vi "SetScanParams.vi"(6 "ScanFunc":i32, 7 "DescKword":string, 8 "error in":errorcluster, 9 "Experiment.lvclass":refnum<class "Experiment.lvclass">, 10 "SinglePar":bool, 11 "Interface.lvclass":refnum<class "Interface.lvclass">) -> (0 "error out":errorcluster, 1 "Experiment.lvclass Out":refnum<class "Experiment.lvclass">, 2 "DataFileName":path, 3 "Interface.lvclass Out":refnum<class "Interface.lvclass">, 4 "Scan list":string[](array[string]), 5 "DataFileRef":refnum<file>)   [LabVIEW 2019, in "Interface.lvclass"]
doc: "Ce Vi prend les données d'acquisition et les formatte en tableau de \"string\" pour ensuite les sauvegarder sous le format .txt"
uses:
  Interface.lvclass
  Experiment Class/Experiment.lvclass
  Interface.lvclass/Interface.ctl
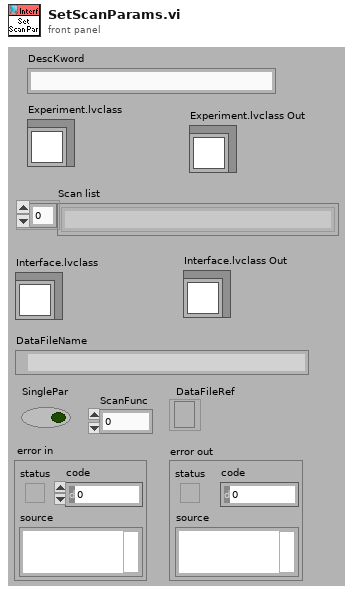
[diagram p1: front panel]
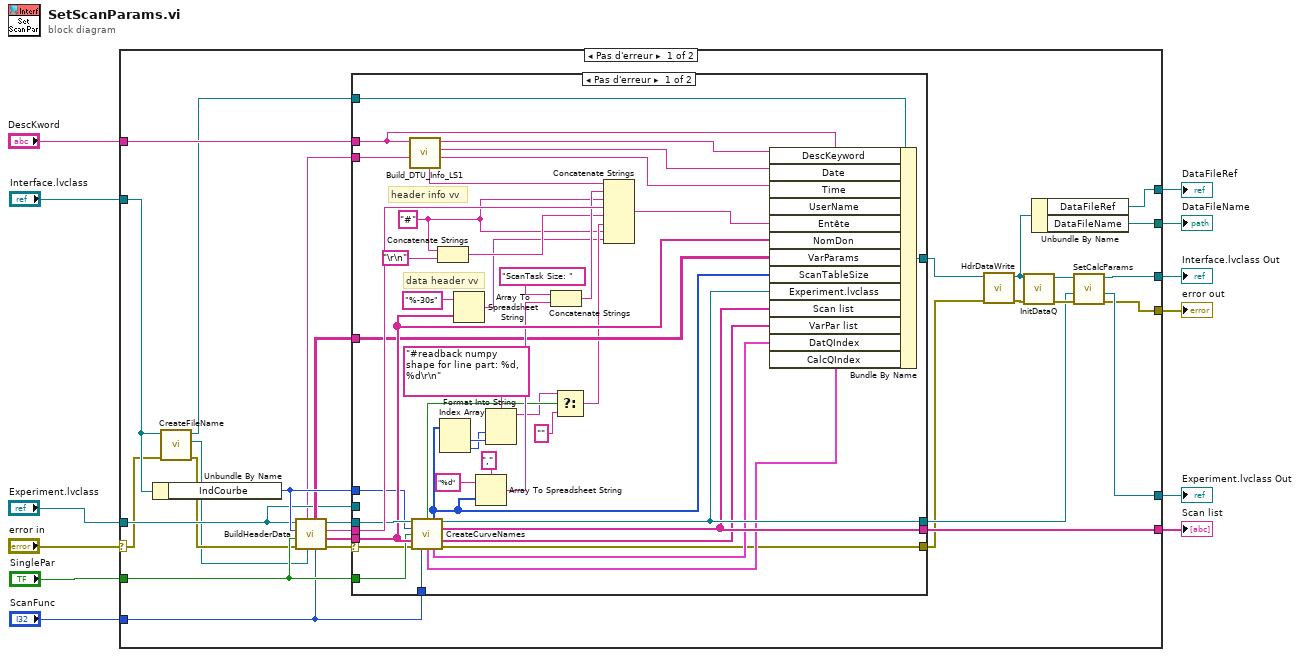
[diagram p0: block diagram]
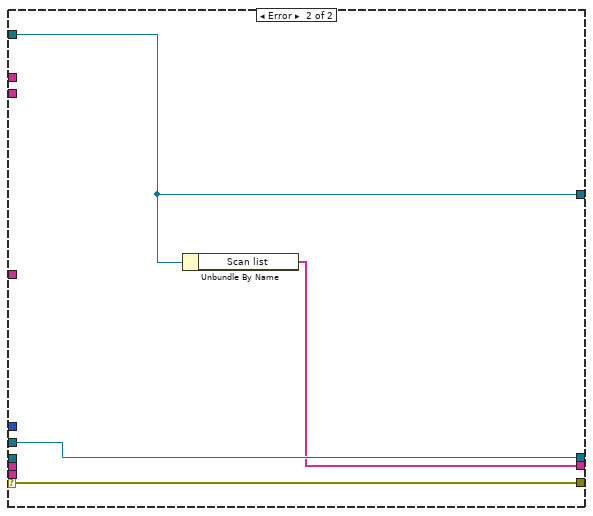
[diagram p2: hidden frame]
diagram:
  n1 = case shown="Pas d'erreur" "error in" {
    selector: "error in" -> [w16 w89]
    tunnel: [w23 w89] -> w12
    tunnel: [w34 w88] -> w9
    tunnel: "Interface.lvclass" -> [w17 w88]
    tunnel: [w39 _] -> w8
    tunnel: [w30 _] -> w7
    tunnel: [w25 _] -> w6
    tunnel: "Experiment.lvclass" -> [w21 w87]
    tunnel: [w31 w87] -> w4
    tunnel: "ScanFunc" -> [w27 _]
    tunnel: "SinglePar" -> [w28 _]
    tunnel: "DescKword" -> [w24 _]
    frame No Error {
      n2 = Unbundle By Name(w17) -> ("IndCourbe"=w36:i64)
      n3 = call "CreateFileName.vi"("error in (no error)"=w16, "Interface.lvclass"=w17) -> ("error out"=w15:errorcluster, "chemin Data"=w13:path, "Interface.lvclass Out"=w14:refnum<class "Interface.lvclass">)  [unwired: 7 in]
      n4 = call "BuildHeaderData.vi"("ScanFunc"=w27, "chemin Data"=w13, "error in"=w15, "SinglePar"=w28, "IndCourbe"=w36, "Experiment.lvclass In"=w21) -> ("error out"=w22:errorcluster, "NomDon"=w38:string[], "HeaderPar"=w41:string, "Experiment.lvclass Out"=w40:refnum<class "Experiment.lvclass">, "VarParams"=w29:string[][], "Experiment Name"=w20:string)
      n5 = case shown="Pas d'erreur" w22 {
        selector: w22 -> [w56 w85]
        tunnel: w41 -> [w82 _]
        tunnel: w40 -> [w81 _]
        tunnel: [w80 w84] -> w18
        tunnel: w38 -> [w78 _]
        tunnel: w36 -> [w77 _]
        tunnel: [w72 w86] -> w32
        tunnel: [w71 w83] -> w30
        tunnel: w29 -> [w67 _]
        tunnel: w14 -> [w66 w84]
        tunnel: w28 -> [w65 _]
        tunnel: w27 -> [w64 _]
        tunnel: [w63 w85] -> w19
        tunnel: w24 -> [w57 _]
        tunnel: w21 -> [_ w86]
        tunnel: w20 -> [w42 _]
        frame No Error {
          w43 = "#" ("chaîne")
          # "data header vv"
          # "header info vv"
          n6 = call "Build_DTU_Info_LS1.vi"("Experiment Path"=w42, "DescKword"=w57) -> ("ScanParUser"=w59:string, "ScanParTime"=w60:string, "ScanParDate"=w61:string, "DTU_HdrStr"=w62:string)  [unwired: 3 in, 3 out]
          n7 = call "CreateCurveNames.vi"("Exp.lvclass In"=w81, "IndCourbe"=w77, "SinglePar"=w65, "NomDon"=w78, "error in"=w56, "ScanFunc"=w64) -> ("MultiScan"=w48:bool, "ScanTableSize"=w53:i32[], "Experiment.lvclass Out"=w72:refnum<class "Experiment.lvclass">, "Scan list"=w71:string[], "VarPar list"=w70:string[], "CalcQIndex"=w68:cluster{"Tableau":i32[]}[], "DataQIndex"=w69:cluster{"Tableau":i32[]}[], "error out"=w63:errorcluster)  [unwired: 2 in]
          n8 = Concatenate Strings(w43, "\r\n") -> (w49:string)
          n9 = Index Array(array=w53) -> (element #1=w52:i32, element #2=w51:i32)  [unwired: 2 in]
          n10 = Array To Spreadsheet String(array=w78, 3:"%-30s" ("format string")) -> (spreadsheet string=w44:string)  [unwired: 1 in]
          n11 = Array To Spreadsheet String(delimiter (Tab)="," ("séparateur (Tabulation)"), array=w53, 3:"%d" ("chaîne de format")) -> (spreadsheet string=w74:string)
          n12 = Format Into String(format string="#readback numpy shape for line part: %d, %d\r\n" ("chaîne"), w51, w52) -> (resulting string=w47:string)  [unwired: 2 in, 1 out]
          n13 = Concatenate Strings("ScanTask Size: " ("chaîne"), w74) -> (w55:string)
          n14 = Select(t=w47, s=w48, f="" ("cas faux")) -> (s? t:f=w45:string)
          n15 = Concatenate Strings(w62, w55, w43, w82, w49, w45, w43, w44) -> (w58:string)
          n16 = Bundle By Name(cluster=w66, "DescKeyword"=w57, "Date"=w61, "Time"=w60, "UserName"=w59, "Entête"=w58, "NomDon"=w78, "VarParams"=w67, "ScanTableSize"=w53, "Experiment.lvclass"=w72, "Scan list"=w71, "VarPar list"=w70, "DatQIndex"=w69, "CalcQIndex"=w68) -> (w80:refnum<class "Interface.lvclass">)
        }
        frame Error {
          n17 = Unbundle By Name(w84) -> ("Scan list"=w83:string[])
        }
      }
      n18 = call "HdrDataWrite.vi"("error in (no error)"=w19, "Interface.lvclass"=w18) -> ("error out"=w37:errorcluster, "Interface.lvclassOut"=w26:refnum<class "Interface.lvclass">)  [unwired: 8 in]
      n19 = call "InitDataQ.vi"("ErrorIn(No Error)"=w37, "Interface.lvclass"=w26) -> ("sortie d'erreur"=w33:errorcluster, "Interface.lvclass Out"=w35:refnum<class "Interface.lvclass">)  [unwired: 8 in]
      n20 = Unbundle By Name(w26) -> ("DataFileRef"=w25:refnum<file>, "DataFileName"=w39:path)
      n21 = call "SetCalcParams.vi"("error in"=w33, "Experiment.lvclass"=w32, "Interface.lvclass"=w35) -> ("error out"=w23:errorcluster, "Experiment.lvclass Out"=w31:refnum<class "Experiment.lvclass">, "Interface.lvclass Out"=w34:refnum<class "Interface.lvclass">)  [unwired: 6 in]
    }
    frame Error {
    }
  }
  "error out" <- w12
  "Interface.lvclass Out" <- w9
  "DataFileName" <- w8
  "Scan list" <- w7
  "DataFileRef" <- w6
  "Experiment.lvclass Out" <- w4
